vi "repPrepareKickoffEnemyPlay.vi"(8 "error in (no error)":errorcluster, 9 "Game in 2":refnum<class "Game.lvclass">, 10 "RobotPlacement":T1(array[cluster]), 11 "PrepareKickoffEnemyPlay in":refnum<class "PrepareKickoffEnemyPlay.lvclass">) -> (0 "error out":errorcluster, 2 "RobotPlacement 2":T1(array[cluster]), 3 "PrepareKickoffEnemyPlay out":refnum<class "PrepareKickoffEnemyPlay.lvclass">)   [LabVIEW 2023, in "PrepareKickoffEnemyPlay.lvclass"]
uses:
  PrepareKickoffEnemyPlay.lvclass
  Game_class/Game.lvclass
  Game_class/Game.lvclass/Game.ctl
  Game_class/Read FieldRef.vi
  Field_class/Field.lvclass
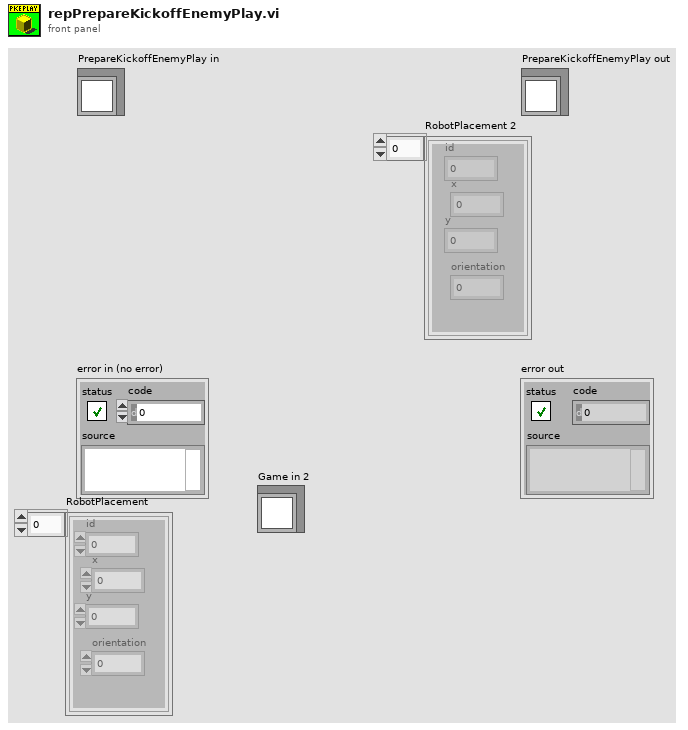
[diagram p1: front panel]
types:
  T1 = cluster{"id":i32, "x":dbl, "y":dbl, "orientation":dbl}[]
  T2 = cluster{"id":i32, "x":dbl, "y":dbl, "orientation":dbl}
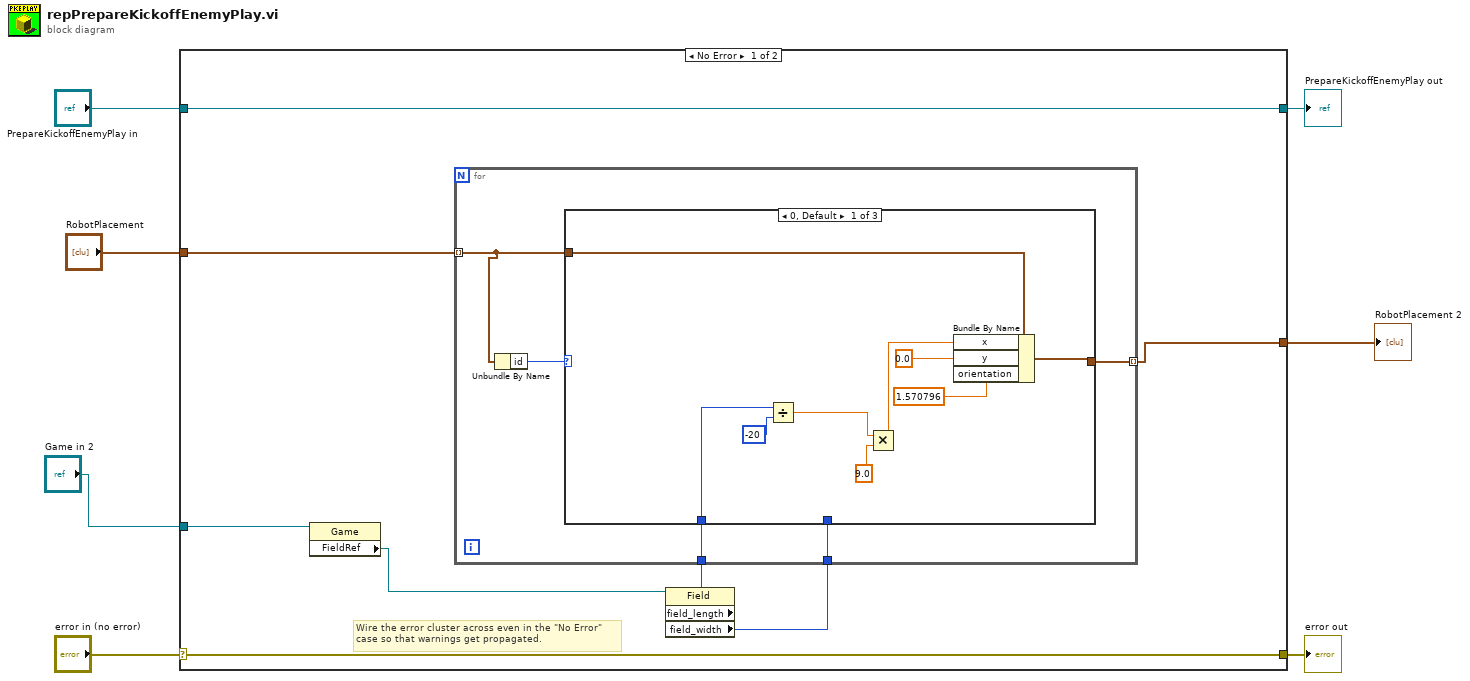
[diagram p0: block diagram]
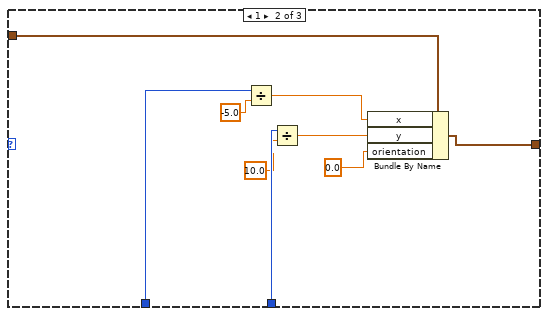
[diagram p2: hidden frame]
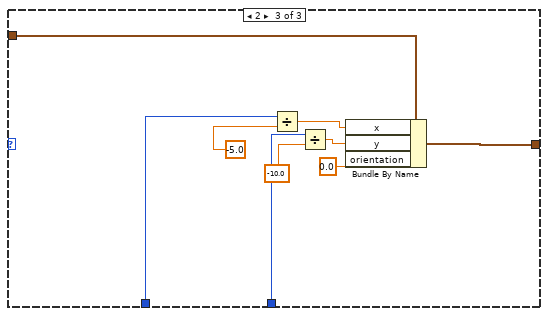
[diagram p3: hidden frame]
diagram:
  n1 = case shown="No Error" "error in (no error)" {
    selector: "error in (no error)" -> [w14 w49]
    tunnel: [w14 w49] -> w6
    tunnel: [w15 w48] -> w4
    tunnel: "PrepareKickoffEnemyPlay in" -> [w15 w48]
    tunnel: [w11 _] -> w3
    tunnel: "RobotPlacement" -> [w10 _]
    tunnel: "Game in 2" -> [w9 _]
    frame No Error {
      # "Wire the error cluster across even in the \"No Error\"\ncase so that warnings get propagated."
      n2 = property class="Game"(reference=w9) -> ("FieldRef"=w8:refnum<class "Field.lvclass">)  [unwired: 1 in, 2 out]
      n3 = property class="Field"(reference=w8) -> ("field_length"=w13:i32, "field_width"=w12:i32)  [unwired: 1 in, 2 out]
      n4 = for {
        tunnel: [w20] -> w11 mode=indexing
        tunnel: w13 -> [w16]
        tunnel: w12 -> [w19]
        tunnel: w10 -> [w18] mode=indexing
        n5 = Unbundle By Name(w18) -> ("id"=w17:i32)
        n6 = case shown="0, Default" w17 {
          tunnel: [w29 w37 w47] -> w20
          tunnel: w19 -> [_ w36 w43]
          tunnel: w18 -> [w25 w31 w40]
          tunnel: w16 -> [w24 w30 w39]
          frame 0, Default {
            n7 = Divide(x=w24, y=-20) -> (x/y=w23:dbl)
            n8 = Multiply(x=w23, y=9.0) -> (x*y=w22:dbl)
            n9 = Bundle By Name(cluster=w25, "x"=w22, "y"=0.0, "orientation"=1.570796) -> (w29:T2)
          }
          frame 1 {
            n10 = Divide(x=w30, y=-5.0 ("x")) -> (x/y=w32:dbl)
            n11 = Divide(x=w36, y=10.0 ("x")) -> (x/y=w33:dbl)
            n12 = Bundle By Name(cluster=w31, "x"=w32, "y"=w33, "orientation"=0.0 ("x")) -> (w37:T2)
          }
          frame 2 {
            n13 = Divide(x=w39, y=-5.0 ("x")) -> (x/y=w41:dbl)
            n14 = Divide(x=w43, y=-10.0 ("x")) -> (x/y=w42:dbl)
            n15 = Bundle By Name(cluster=w40, "x"=w41, "y"=w42, "orientation"=0.0) -> (w47:T2)
          }
        }
      }
    }
    frame Error {
    }
  }
  "error out" <- w6
  "PrepareKickoffEnemyPlay out" <- w4
  "RobotPlacement 2" <- w3
